vi "Get Perform Action Strategy.vi"(11 "Virtual Instrument in":refnum<class "Virtual Instrument.lvclass">) -> (2 "Perform Action Strategy":refnum<class "Perform Action Strategy.lvclass">, 3 "Virtual Instrument out":refnum<class "Virtual Instrument.lvclass">)   [LabVIEW 2023, in "HAL.lvlib" / "Virtual Instrument.lvclass"]
uses:
  Virtual Instrument.lvclass
  Virtual Instrument.lvclass/Virtual Instrument.ctl
  Perform Action Strategy/Perform Action Strategy.lvclass
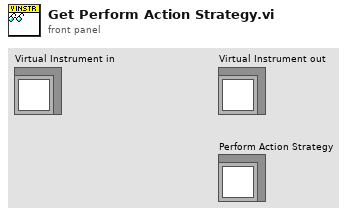
[diagram p1: front panel]
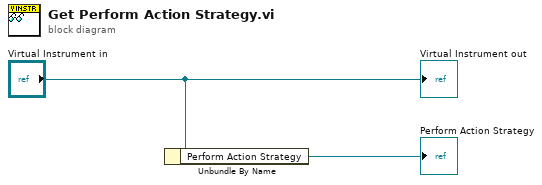
[diagram p0: block diagram]
diagram:
  n1 = Unbundle By Name("Virtual Instrument in") -> ("Perform Action Strategy"=→"Perform Action Strategy":refnum<class "Perform Action Strategy.lvclass">)
  "Virtual Instrument out" <- "Virtual Instrument in"
